vi "DataINI.vi"(8 "error in (no error)":errorcluster caption="错误输入（无错误）", 11 "MainPage 输入":refnum<class "MainPage.lvclass">) -> (0 "error out":errorcluster caption="错误输出", 3 "MainPage 输出":refnum<class "MainPage.lvclass">)   [LabVIEW 2019, in "MainPage.lvlib" / "MainPage.lvclass"]
uses:
  MainPage.lvclass
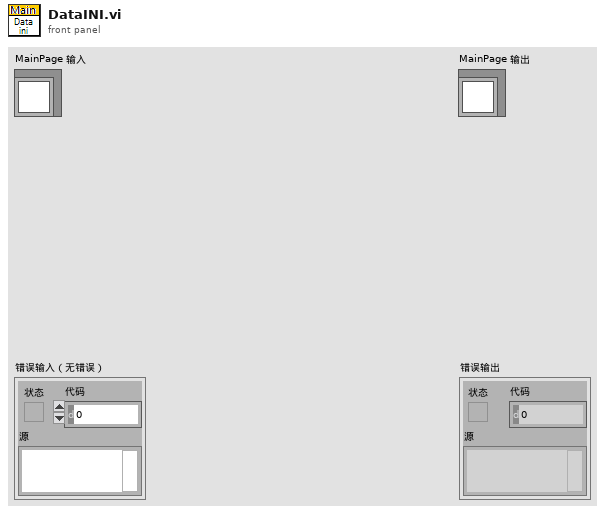
[diagram p1: front panel]
types:
  T1 = enum16{"ini", "增加记录", "读取记录", "更改寄存器值", "更改接口状态", "更改报文信息", "增加报文信息"}
  T2 = enum16{"ini", "读取", "写入-报文记录", "写入-寄存器模拟", "写入-串口状态", "增加报文记录"}
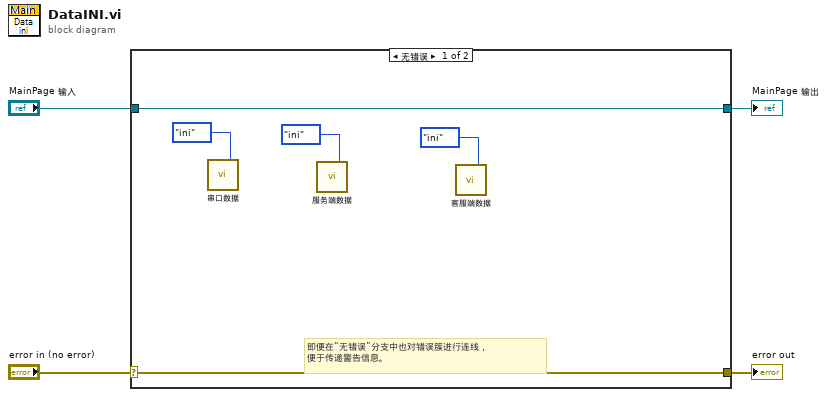
[diagram p0: block diagram]
diagram:
  n1 = case shown="无错误" "error in (no error)" {
    selector: "error in (no error)" -> [w8 w11]
    tunnel: [w8 w11] -> w3
    tunnel: [w9 w10] -> w1
    tunnel: "MainPage 输入" -> [w9 w10]
    frame No Error {
      # "即便在“无错误”分支中也对错误簇进行连线，\n便于传递警告信息。"
      n2 = call "串口数据.vi"("枚举"=T2."ini") -> ()  [unwired: 18 in, 1 out]
      n3 = call "服务端数据.vi"("枚举"=T1."ini") -> ()  [unwired: 17 in, 2 out]
      n4 = call "客服端数据.vi"("枚举"=T1."ini") -> ()  [unwired: 17 in, 2 out]
    }
    frame Error {
    }
  }
  "error out" <- w3
  "MainPage 输出" <- w1
